vi "CRYDrop Data in Same Graph.vi"(4 "pGraph VI":refnum<vi>, 6 "Queue":refnum<queue>, 7 "Total Plot In":u32, 11 "sAction":string) -> (2 "Accepted?":bool, 3 "Total Plot Out":u32)   [LabVIEW 2013]
uses:
  CRYData View Global.vi
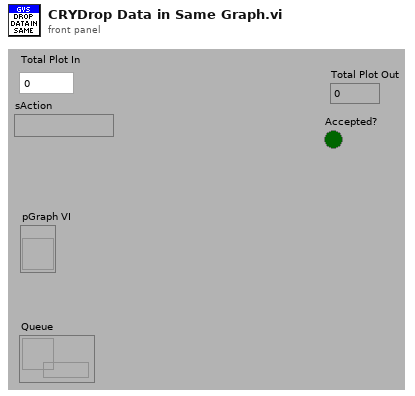
[diagram p1: front panel]
types:
  T1 = typedef "CRYDrag Graph.ctl" = cluster{"GraphType":string, "GraphData":variant}
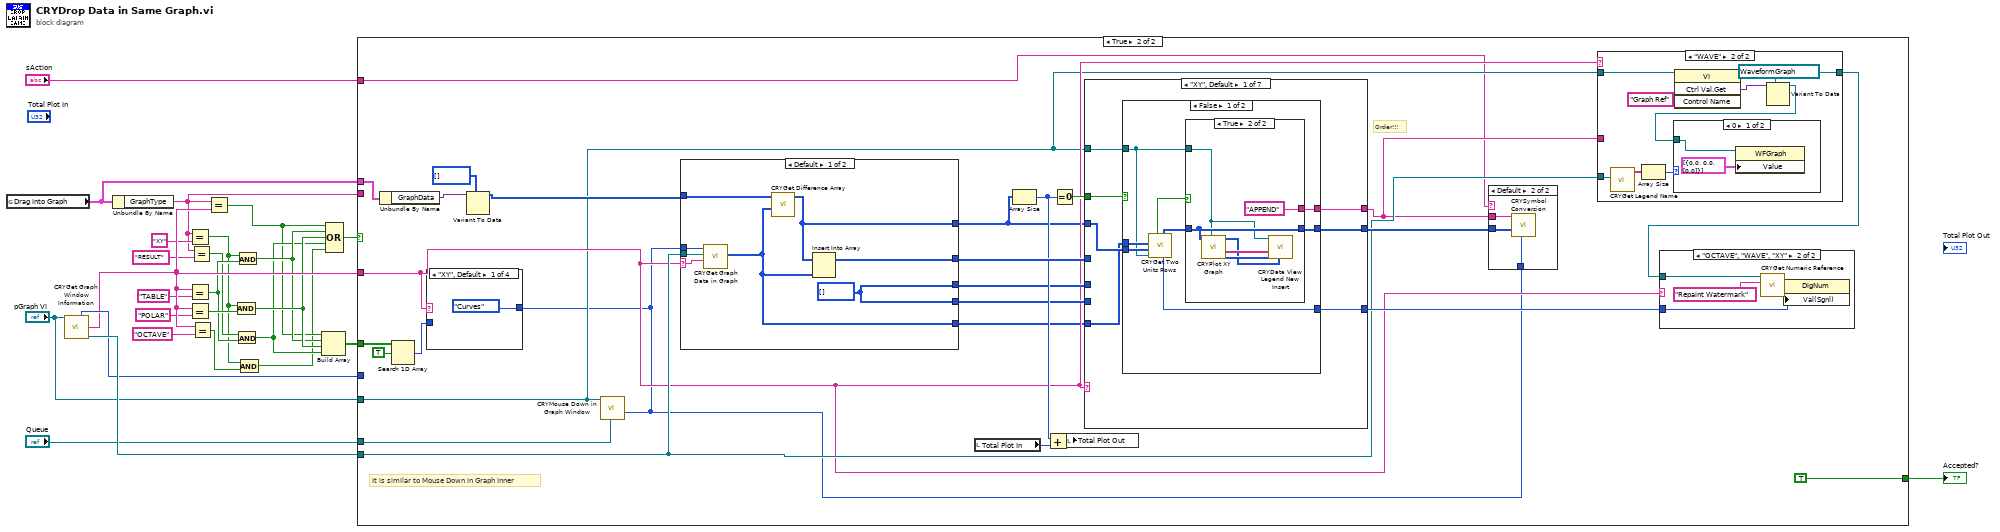
[diagram p0: block diagram]
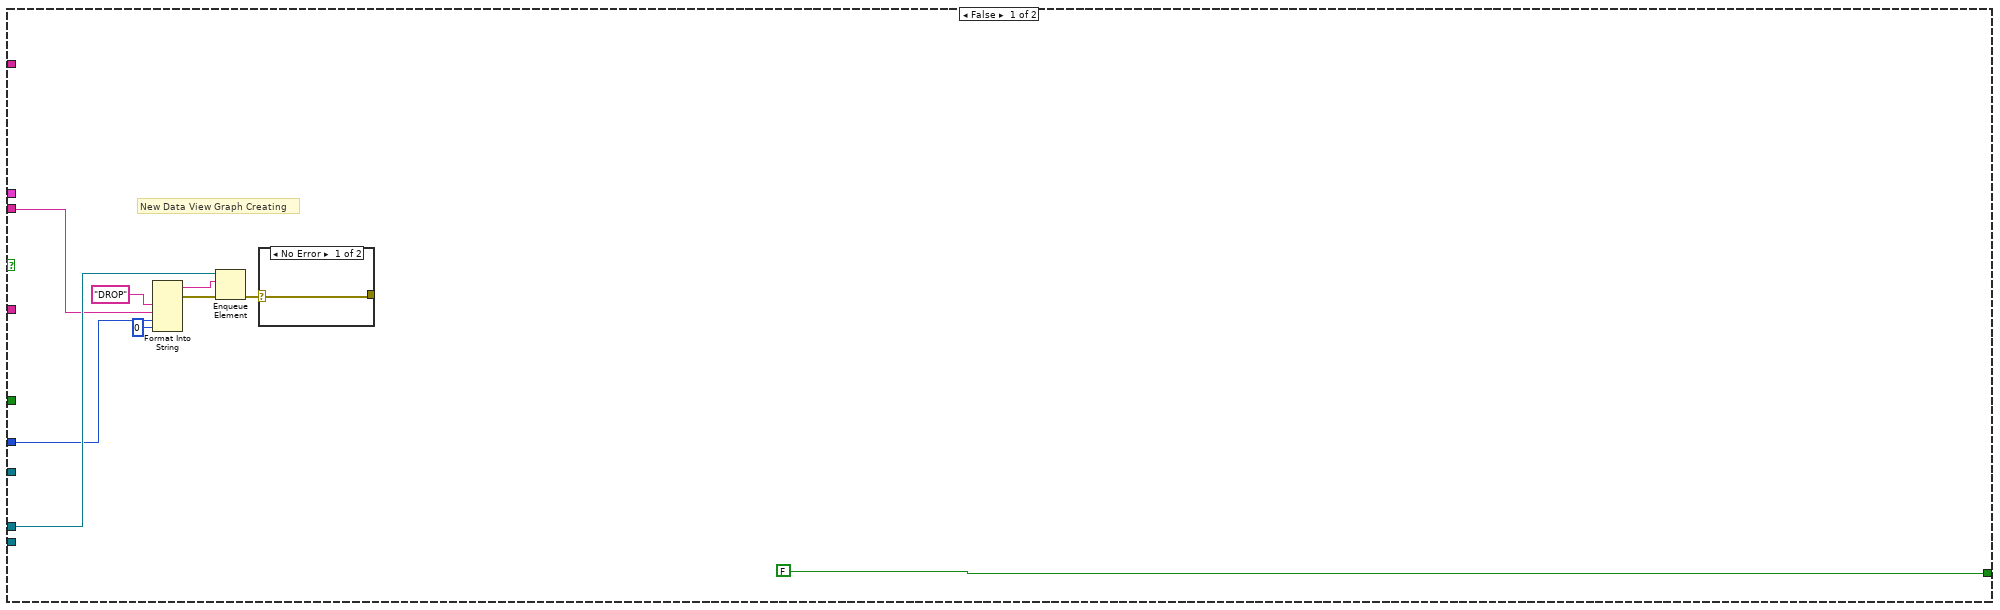
[diagram p2: hidden frame]
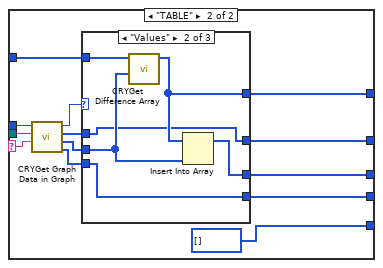
[diagram p8: hidden frame]
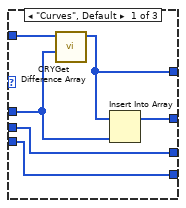
[diagram p9: hidden frame]
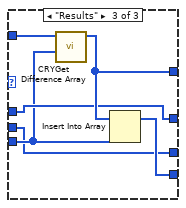
[diagram p10: hidden frame]
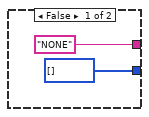
[diagram p11: hidden frame]
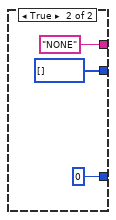
[diagram p12: hidden frame]
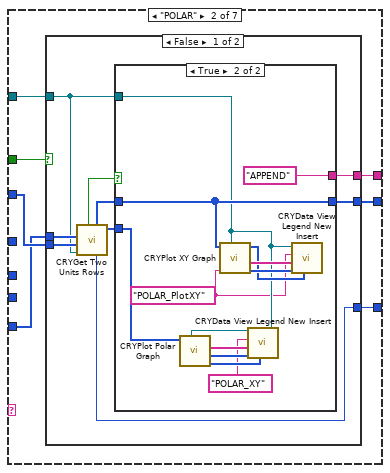
[diagram p13: hidden frame]
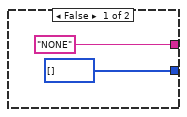
[diagram p14: hidden frame]
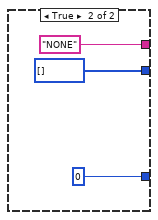
[diagram p15: hidden frame]
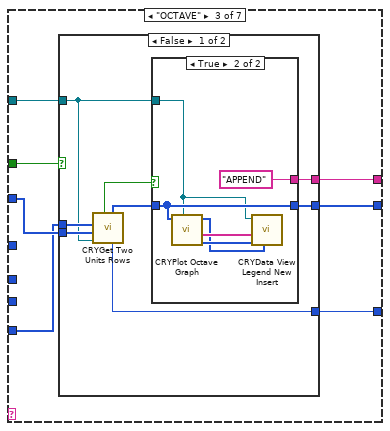
[diagram p16: hidden frame]
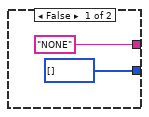
[diagram p17: hidden frame]
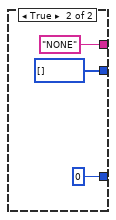
[diagram p18: hidden frame]
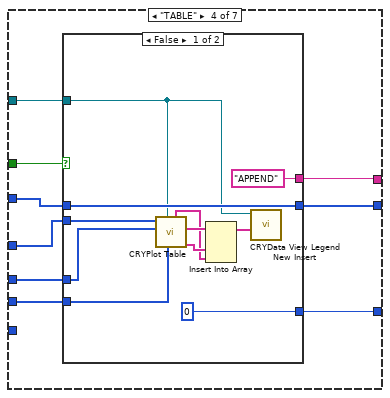
[diagram p19: hidden frame]
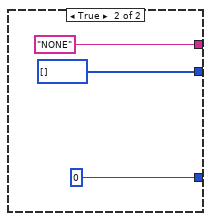
[diagram p20: hidden frame]
diagram:
  n1 = global read "CRYData View Global.vi" "Drag into Graph"() -> (w20:T1)
  n2 = call "CRYGet Graph Window Information.vi"("pGraph VI In"="pGraph VI") -> ("Graph Number Out"=w24:i32, "Graph Type Out"=w22:string, "Legend Ref Out"=w25:refnum<vi>)  [unwired: 4 in, 8 out]
  n3 = Unbundle By Name(w20) -> ("GraphType"=w11:string)
  n4 = Equal?(x=w11, y="XY") -> (x = y?=w4:bool)
  n5 = Equal?(x=w22, y="TABLE") -> (x = y?=w6:bool)
  n6 = Equal?(x=w22, y="POLAR") -> (x = y?=w15:bool)
  n7 = Equal?(x=w11, y="RESULT") -> (x = y?=w5:bool)
  n8 = Equal?(x=w22, y="OCTAVE") -> (x = y?=w3:bool)
  n9 = Equal?(x=w11, y=w22) -> (x = y?=w8:bool)
  n10 = Compound Arithmetic op=AND(w4, w15) -> (w14:bool)
  n11 = Compound Arithmetic op=AND(w5, w6) -> (w9:bool)
  n12 = Compound Arithmetic op=AND(w4, w6) -> (w13:bool)
  n13 = Compound Arithmetic op=AND(w4, w3) -> (w2:bool)
  n14 = Build Array(w8, w13, w14, w9) -> (w12:bool[])
  n15 = Compound Arithmetic op=OR(w8, w13, w14, w9, w2) -> (w18:bool)
  n16 = case shown="True" w18 {
    tunnel: [FALSE TRUE] -> w26
    tunnel: "Queue" -> [w34 w58]
    tunnel: w22 -> [_ w43]
    tunnel: w20 -> [_ w62]
    tunnel: w11 -> [w33 _]
    tunnel: w12 -> [_ w61]
    tunnel: w24 -> [w32 _]
    tunnel: w25 -> [_ w48]
    tunnel: "pGraph VI" -> [_ w42]
    tunnel: "sAction" -> [_ w38]
    frame False {
      # "New Data View Graph Creating"
      n17 = Format Into String("DROP" ("input 1"), w33, w32, 0 ("input 4")) -> (resulting string=w30:string, error out=w28:errorcluster)  [unwired: 3 in]
      n18 = Enqueue Element(queue=w34, element=w30, error in (no error)=w28) -> (error out=w27:errorcluster)  [unwired: 3 out]
      n19 = case shown="No Error" w27 {
        selector: w27 -> [w36 w37]
        tunnel: [w36 w37] -> _
        frame No Error {
        }
        frame Error {
        }
      }
    }
    frame True {
      # "Order!!!"
      # "It is similar to Mouse Down in Graph Inner"
      n20 = Unbundle By Name(w62) -> ("GraphData"=w63:variant)
      n21 = Search 1D Array(1D array=w61, element=TRUE) -> (index of element=w59:i32)  [unwired: 1 in]
      n22 = case shown="\"XY\", Default" w43 {
        tunnel: [enum16{"Curves", "Values", "Results", "WFM"}."Curves" ("Type") w294 enum16{"Curves", "Values", "Results", "WFM"}."Results" ("Type") enum16{"Curves", "Values", "Results", "WFM"}."WFM" ("Type")] -> w41
        tunnel: w59 -> [_ w293 _ _]
        frame "XY", Default {
        }
        frame "TABLE" {
          n23 = case shown="Default" w293 {
            tunnel: [enum16{"Curves", "Values", "Results", "WFM"}."Curves" ("Type") enum16{"Curves", "Values", "Results", "WFM"}."Results" ("Type") enum16{"Curves", "Values", "Results", "WFM"}."Values" ("Type")] -> w294
            frame 1 {
            }
            frame 3 {
            }
            frame Default {
            }
          }
        }
        frame "RESULT" {
        }
        frame "WAVE" {
        }
      }
      n24 = Variant To Data(type=i32[] [] ("Drag Rows"), Variant=w63) -> (data=w44:i32[])  [unwired: 1 in, 1 out]
      n25 = call "CRYMouse Down in Graph Window.vi"("Queue"=w58, "Selected Type"=w41, "pGraph VI In"=w42) -> ()  [unwired: 8 in, 1 out]
      n26 = case shown="Default" w43 {
        selector: w43 -> [w85 w98]
        tunnel: w48 -> [w91 w104]
        tunnel: w44 -> [w90 w103]
        tunnel: [w89 w102] -> w54
        tunnel: [w88 w101] -> w40
        tunnel: w41 -> [w87 w100]
        tunnel: [w86 i32[] [] ("Rows")] -> w39
        tunnel: [w84 w94] -> w51
        tunnel: [w84 w93] -> w50
        frame Default {
          w84 = i32[] [] ("Value Rows")
          n27 = call "CRYGet Graph Data in Graph.vi"("Graph Type"=w85, "Legend Refnum"=w91, "Type In"=w87) -> ("Rows"=w86:i32[])  [unwired: 1 in, 7 out]
          n28 = call "CRYGet Difference Array.vi"("Array 2"=w86, "Array 1"=w90) -> ("Diff Out"=w88:i32[])  [unwired: 3 in, 6 out]
          n29 = Insert Into Array(array=w88, new element=w86) -> (w89:i32[])  [unwired: 1 in]
        }
        frame "TABLE" {
          n30 = call "CRYGet Graph Data in Graph.vi"("Graph Type"=w98, "Legend Refnum"=w104, "Type In"=w100) -> ("Result Rows"=w96:i32[], "Value Rows"=w97:i32[], "Rows"=w99:i32[], "Type Out"=w95:enum16{"Curves", "Values", "Results", "WFM"})  [unwired: 1 in, 4 out]
          n31 = case shown="\"Values\"" w95 {
            tunnel: w103 -> [w110 w116 w122]
            tunnel: [w109 w112 w120] -> w102
            tunnel: [w108 w115 w121] -> w101
            tunnel: w99 -> [w107 w112 w120]
            tunnel: w97 -> [w106 w114 w117]
            tunnel: w96 -> [w105 w111 w119]
            tunnel: [w106 w113 w117] -> w94
            tunnel: [w105 w111 w118] -> w93
            frame "Curves", Default {
              n32 = call "CRYGet Difference Array.vi"("Array 2"=w107, "Array 1"=w110) -> ("Diff Out"=w108:i32[])  [unwired: 3 in, 6 out]
              n33 = Insert Into Array(array=w108, new element=w107) -> (w109:i32[])  [unwired: 1 in]
            }
            frame "Values" {
              n34 = call "CRYGet Difference Array.vi"("Array 2"=w114, "Array 1"=w116) -> ("Diff Out"=w115:i32[])  [unwired: 3 in, 6 out]
              n35 = Insert Into Array(array=w115, new element=w114) -> (w113:i32[])  [unwired: 1 in]
            }
            frame "Results" {
              n36 = call "CRYGet Difference Array.vi"("Array 2"=w119, "Array 1"=w122) -> ("Diff Out"=w121:i32[])  [unwired: 3 in, 6 out]
              n37 = Insert Into Array(array=w121, new element=w119) -> (w118:i32[])  [unwired: 1 in]
            }
          }
        }
      }
      n38 = local read "Total Plot In"() -> (w56:u32)
      n39 = Array Size(array=w40) -> (size(s)=w53:i32)
      n40 = Add(x=w53, y=w56) -> (x+y=w55:u32)
      n41 = Equal To 0?(x=w53) -> (x = 0?=w52:bool)
      n42 = local write "Total Plot Out"(w55) -> ()
      n43 = case shown="\"XY\", Default" w43 {
        tunnel: [w129 w155 w188 w216 w237 w253 w280] -> w57
        tunnel: w54 -> [_ _ _ w213 w236 _ _]
        tunnel: w40 -> [w127 w153 w186 w214 w234 w248 w275]
        tunnel: w52 -> [w128 w154 w187 w215 w235 w252 w279]
        tunnel: w39 -> [w126 w152 w185 _ _ w249 w276]
        tunnel: w51 -> [_ _ _ w212 _ _ _]
        tunnel: w50 -> [_ _ _ w211 _ _ _]
        tunnel: [w125 w151 w184 w210 w233 w251 w278] -> w49
        tunnel: [w124 w150 w183 w209 w232 w250 w277] -> w47
        tunnel: w42 -> [w123 w149 w182 w208 w231 w247 w274]
        frame "XY", Default {
          n44 = case shown="False" w128 {
            tunnel: w126 -> [w132 _]
            tunnel: [w137 0 ("Two Units")] -> w129
            tunnel: w127 -> [w131 _]
            tunnel: [w134 i32[] [] ("New Rows Out")] -> w125
            tunnel: [w133 "NONE" ("sActin")] -> w124
            tunnel: w123 -> [w130 _]
            frame False {
              n45 = call "CRYGet Two Units Rows.vi"("pGraph VI In"=w130, "New Rows In"=w131, "Old Rows In"=w132) -> ("Two Units"=w137:i32, "New Rows Out"=w135:i32[], "New Exist?"=w136:bool)  [unwired: 2 in, 4 out]
              n46 = case shown="True" w136 {
                tunnel: w135 -> [_ w142]
                tunnel: [i32[] [] ("New Rows Out") w142] -> w134
                tunnel: ["NONE" ("sActin") "APPEND" ("sActin")] -> w133
                tunnel: w130 -> [_ w140]
                frame False {
                }
                frame True {
                  n47 = call "CRYPlot XY Graph.vi"("pGraph VI In"=w140, "Selected Rows In"=w142) -> ("Color Info"=w144:u32[], "Curve Name"=w145:string[], "ItemSyms"=w141:i32[])  [unwired: 4 in, 3 out]
                  n48 = call "CRYData View Legend New Insert.vi"("Item Symbols"=w141, "Color Array"=w144, "ItemName Array"=w145, "pGraph VI In"=w140) -> ()  [unwired: 7 in, 1 out]
                }
              }
            }
            frame True {
            }
          }
        }
        frame "POLAR" {
          n49 = case shown="False" w154 {
            tunnel: w152 -> [w159 _]
            tunnel: [w164 0 ("Two Units")] -> w155
            tunnel: w153 -> [w158 _]
            tunnel: [w161 i32[] [] ("New Rows Out")] -> w151
            tunnel: [w160 "NONE" ("sActin")] -> w150
            tunnel: w149 -> [w156 _]
            frame False {
              n50 = call "CRYGet Two Units Rows.vi"("pGraph VI In"=w156, "New Rows In"=w158, "Old Rows In"=w159) -> ("All Rows Out"=w157:i32[], "Two Units"=w164:i32, "New Rows Out"=w162:i32[], "New Exist?"=w163:bool)  [unwired: 2 in, 3 out]
              n51 = case shown="True" w163 {
                tunnel: w162 -> [_ w175]
                tunnel: [i32[] [] ("New Rows Out") w175] -> w161
                tunnel: ["NONE" ("sActin") "APPEND" ("sActin")] -> w160
                tunnel: w157 -> [_ w173]
                tunnel: w156 -> [_ w168]
                frame False {
                }
                frame True {
                  w167 = "POLAR_PlotXY" ("sActin")
                  n52 = call "CRYPlot Polar Graph.vi"("pGraph VI In"=w168, "Selected Rows In"=w173) -> ("ItemSyms"=w172:i32[], "Freq Color"=w171:u32[], "Freq Name"=w170:string[])  [unwired: 6 in, 1 out]
                  n53 = call "CRYPlot XY Graph.vi"("pGraph VI In"=w168, "sType"=w167, "Selected Rows In"=w175) -> ("Color Info"=w177:u32[], "Curve Name"=w178:string[], "ItemSyms"=w174:i32[])  [unwired: 3 in, 3 out]
                  n54 = call "CRYData View Legend New Insert.vi"("Item Symbols"=w172, "Color Array"=w171, "ItemName Array"=w170, "sOption"="POLAR_XY" ("sActin"), "pGraph VI In"=w168) -> ()  [unwired: 6 in, 1 out]
                  n55 = call "CRYData View Legend New Insert.vi"("Item Symbols"=w174, "Color Array"=w177, "ItemName Array"=w178, "sOption"=w167, "pGraph VI In"=w168) -> ()  [unwired: 6 in, 1 out]
                }
              }
            }
            frame True {
            }
          }
        }
        frame "OCTAVE" {
          n56 = case shown="False" w187 {
            tunnel: w185 -> [w191 _]
            tunnel: [w196 0 ("Two Units")] -> w188
            tunnel: w186 -> [w190 _]
            tunnel: [w193 i32[] [] ("New Rows Out")] -> w184
            tunnel: [w192 "NONE" ("sActin")] -> w183
            tunnel: w182 -> [w189 _]
            frame False {
              n57 = call "CRYGet Two Units Rows.vi"("pGraph VI In"=w189, "New Rows In"=w190, "Old Rows In"=w191) -> ("Two Units"=w196:i32, "New Rows Out"=w194:i32[], "New Exist?"=w195:bool)  [unwired: 2 in, 4 out]
              n58 = case shown="True" w195 {
                tunnel: w194 -> [_ w201]
                tunnel: [i32[] [] ("New Rows Out") w201] -> w193
                tunnel: ["NONE" ("sActin") "APPEND" ("sActin")] -> w192
                tunnel: w189 -> [_ w199]
                frame False {
                }
                frame True {
                  n59 = call "CRYPlot Octave Graph.vi"("pGraph VI In"=w199, "Selected Rows In"=w201) -> ("Color Info"=w203:u32[], "Curve Name"=w204:string[], "ItemSyms"=w200:i32[])  [unwired: 6 in, 1 out]
                  n60 = call "CRYData View Legend New Insert.vi"("Item Symbols"=w200, "Color Array"=w203, "ItemName Array"=w204, "pGraph VI In"=w199) -> ()  [unwired: 7 in, 1 out]
                }
              }
            }
            frame True {
            }
          }
        }
        frame "TABLE" {
          n61 = case shown="False" w215 {
            tunnel: w213 -> [w226 _]
            tunnel: [0 ("Two Units") 0 ("Two Units")] -> w216
            tunnel: w214 -> [w223 _]
            tunnel: w212 -> [w225 _]
            tunnel: w211 -> [w224 _]
            tunnel: [w223 i32[] [] ("Diff Out")] -> w210
            tunnel: ["APPEND" ("sActin") "NONE" ("sActin")] -> w209
            tunnel: w208 -> [w217 _]
            frame False {
              n62 = call "CRYPlot Table.vi"("Result Rows In"=w224, "pGraph VI In"=w217, "Value Rows In"=w225, "Curve Rows In"=w226) -> ("Value Name"=w220:string[], "Curve Name"=w221:string[], "Result Name"=w219:string[])  [unwired: 2 in, 3 out]
              n63 = Insert Into Array(array=w221, new element #1=w220, new element #2=w219) -> (w218:string[])  [unwired: 1 in]
              n64 = call "CRYData View Legend New Insert.vi"("ItemName Array"=w218, "pGraph VI In"=w217) -> ()  [unwired: 9 in, 1 out]
            }
            frame True {
            }
          }
        }
        frame "RESULT" {
          n65 = case shown="False" w235 {
            tunnel: w236 -> [_ w246]
            tunnel: [0 ("Two Units") 0 ("Two Units")] -> w237
            tunnel: w234 -> [_ w244]
            tunnel: [i32[] [] ("Diff Out") w244] -> w233
            tunnel: ["NONE" ("sActin") "APPEND" ("sActin")] -> w232
            tunnel: w231 -> [_ w241]
            frame True {
            }
            frame False {
              n66 = call "CRYPlot Result.vi"("pGraph VI In"=w241, "Old Rows In"=w246) -> ("Curve Name"=w242:string[])  [unwired: 4 in, 5 out]
              n67 = call "CRYData View Legend New Insert.vi"("ItemName Array"=w242, "pGraph VI In"=w241) -> ()  [unwired: 3 in, 7 out]
            }
          }
        }
        frame "WAVE" {
          n68 = case shown="False" w252 {
            tunnel: [0 ("Two Units") w258] -> w253
            tunnel: [i32[] [] ("Diff Out") w264] -> w251
            tunnel: ["NONE" ("sActin") w265] -> w250
            tunnel: w249 -> [_ w260]
            tunnel: w248 -> [_ w259]
            tunnel: w247 -> [_ w257]
            frame True {
            }
            frame False {
              n69 = call "CRYGet Two Units Rows.vi"("pGraph VI In"=w257, "New Rows In"=w259, "Old Rows In"=w260, "Type"=enum16{"Curves", "Values", "Results", "WFM"}."WFM") -> ("Two Units"=w258:i32, "New Rows Out"=w262:i32[], "New Exist?"=w263:bool)  [unwired: 1 in, 4 out]
              n70 = case shown="True" w263 {
                tunnel: ["NONE" ("sActin") "APPEND" ("sActin")] -> w265
                tunnel: w262 -> [_ w269]
                tunnel: [i32[] [] ("Diff Out") w269] -> w264
                tunnel: w257 -> [_ w268]
                frame False {
                }
                frame True {
                  n71 = call "CRYPlot Wave Graph.vi"("pGraph VI In"=w268, "Selected Rows In"=w269) -> ("ItemSyms"=w270:i32[], "Color Info"=w272:u32[], "Curve Name"=w273:string[])  [unwired: 3 in, 4 out]
                  n72 = call "CRYData View Legend New Insert.vi"("Item Symbols"=w270, "Color Array"=w272, "ItemName Array"=w273, "pGraph VI In"=w268) -> ()  [unwired: 7 in, 1 out]
                }
              }
            }
          }
        }
        frame "INTENSITY" {
          n73 = case shown="True" w279 {
            tunnel: [0 ("Two Units") _] -> w280
            tunnel: [i32[] [] ("Diff Out") w285] -> w278
            tunnel: ["NONE" ("sActin") "APPEND" ("sActin")] -> w277
            tunnel: w276 -> [_ w287]
            tunnel: w275 -> [_ w286]
            tunnel: w274 -> [_ w284]
            frame True {
            }
            frame False {
              n74 = Insert Into Array(array=w287, new element=w286) -> (w285:i32[])  [unwired: 1 in]
              n75 = call "CRYPlot Intensity Graph.vi"("pGraph VI In"=w284, "Selected Rows In"=w285) -> ("ItemSyms"=w288:i32[], "Color Info"=w289:u32[], "Wave Names"=w290:string[])  [unwired: 6 in, 1 out]
              n76 = call "CRYData View Legend New Insert.vi"("Item Symbols"=w288, "Color Array"=w289, "ItemName Array"=w290, "pGraph VI In"=w284) -> ()  [unwired: 7 in, 1 out]
            }
          }
        }
      }
      n77 = case shown="Default" w38 {
        tunnel: w49 -> [_ w67]
        tunnel: w47 -> [_ w66]
        tunnel: w41 -> [_ w65]
        frame "ViewReport" {
        }
        frame Default {
          n78 = call "CRYSymbol Conversion.vi"("CurLib Tab Type"=w65, "nDatas"=w67, "sActin"=w66) -> ()  [unwired: 9 in]
        }
      }
      n79 = case shown="\"WAVE\"" w43 {
        tunnel: w48 -> [_ w75]
        tunnel: w42 -> [w68 w71]
        tunnel: w47 -> [_ _]
        tunnel: [w68 w69] -> w46
        frame "False", Default {
        }
        frame "WAVE" {
          n80 = call "CRYGet Legend Name.vi"("MCListbox Refnum"=w75) -> ("Names Out"=w76:string[])  [unwired: 2 in, 8 out]
          n81 = Array Size(array=w76) -> (size(s)=w77:i32)
          n82 = invoke class="VI" method="Ctrl Val.Get"(reference=w71, "Control Name"="Graph Ref") -> (reference out=w69:refnum<vi>, "Get Control Value Variant"=w72:variant)  [unwired: 2 in, 2 out]
          n83 = Variant To Data(type=refnum<vi> refnum ("WaveGraph Ref"), Variant=w72) -> (data=w70:refnum<vi>)  [unwired: 1 in, 1 out]
          n84 = case shown="0" w77 {
            tunnel: w70 -> [w79 _]
            frame 0 {
              n85 = property class="WFGraph"(reference=w79, "Value"=cluster{"xo":dbl, "dx":dbl, dbl[]}[] [{"xo"=0.0, "dx"=0.0, [0.0]}] ("appended array")) -> ()  [unwired: 1 in, 2 out]
            }
            frame 1, Default {
            }
          }
        }
      }
      n86 = case shown="\"OCTAVE\", \"WAVE\", \"XY\"" w43 {
        tunnel: w46 -> [_ w81]
        tunnel: w57 -> [_ w80]
        frame Default {
        }
        frame "OCTAVE", "WAVE", "XY" {
          n87 = call "CRYGet Numeric Reference.vi"("Label Name"="Repaint Watermark" ("Control Name"), "VI Refnum"=w81) -> ("Numeric Ref Out"=w83:refnum<vi>)  [unwired: 9 out]
          n88 = property class="DigNum"(reference=w83, "Val(Sgnl)"=w80) -> ()  [unwired: 1 in, 2 out]
        }
      }
    }
  }
  "Accepted?" <- w26
